vi "20211015_02.vi"() -> ()   [LabVIEW 2019]
panel:
  out "String C":string
  in  "String B":string
  in  "String A":string
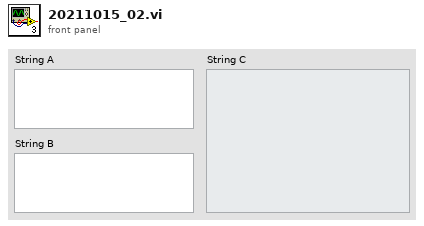
[diagram p1: front panel]
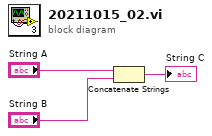
[diagram p0: block diagram]
diagram:
  n1 = Concatenate Strings("String A", "String B") -> (→"String C":string)
